vi "VerificarStop.vi"(7 "error in":errorcluster, 10 "Notifier in":refnum<notifier>) -> (0 "error out":errorcluster, 2 "stop":bool, 3 "Notifier out":refnum<notifier>)   [LabVIEW 2015]
uses:
  Login Window Control Folder/EnumEstado.ctl
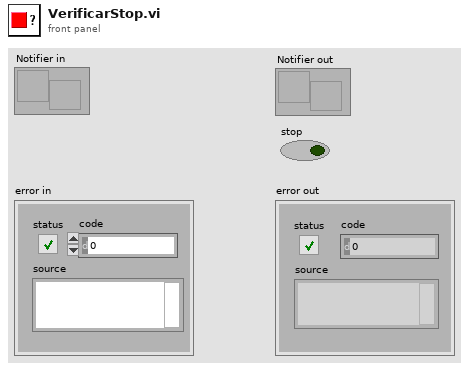
[diagram p1: front panel]
types:
  T1 = typedef "EnumEstado.ctl" = enum16{"Stop", "Iniciado", "Log In", "Log Out", "Escribir", "Leer Radiacion", "Leer Temp", "Leer Humed Relat", "Leer Temp del Panel", "Leer Pot Panel", "Leer Pot Fase R", "Leer Pot Fase  S", "Leer PotFase T", "Leer Nivel Bat", "Leer Pot Generador"}
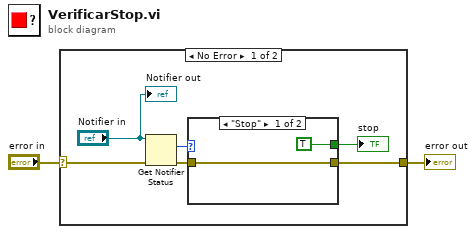
[diagram p0: block diagram]
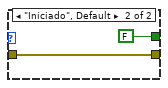
[diagram p2: hidden frame]
diagram:
  n1 = case shown="No Error" "error in" {
    selector: "error in" -> [w3 w13]
    tunnel: [w4 w13] -> w2
    frame No Error {
      n2 = Get Notifier Status(notifier="Notifier in", error in (no error)=w3) -> (current notification=w7:T1, error out=w5:errorcluster)  [unwired: 3 out]
      n3 = case shown="\"Stop\"" w7 {
        tunnel: [TRUE FALSE] -> w8
        tunnel: w5 -> [w9 w11]
        tunnel: [w9 w11] -> w4
        frame "Stop" {
        }
        frame "Iniciado", Default {
        }
      }
      "stop" <- w8
      "Notifier out" <- "Notifier in"
    }
    frame Error {
    }
  }
  "error out" <- w2
